vi "DepthSense Acquire.vi"(8 "error in (no error)":errorcluster) -> (0 "error out":errorcluster, 3 "new depth frame":T1)   [LabVIEW 2011]
uses:
  <vilib>/vision/Image Controls.llb/IMAQ Image.ctl
  IT WORKS SO SUCK IT/DepthSense Global Status.vi
  <vilib>/vision/NI_Vision_Development_Module.lvlib
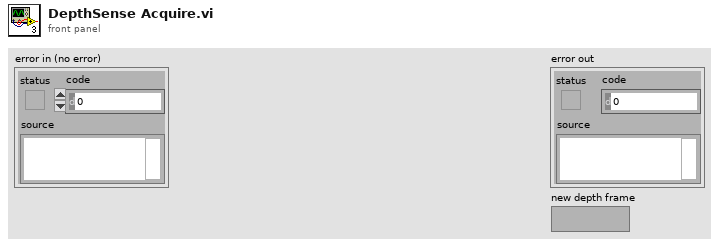
[diagram p1: front panel]
types:
  T1 = typedef "IMAQ Image.ctl" = refnum<image>
  T2 = typedef "Image Type" = u32
  T3 = cluster{"Camera Version":string, "Image Height":i32, "Image Width":i32, "Minimum Framerate":i32, "Maximum Framerate":i32, "Framerate":i32, "Close Mode":bool, "Denoising":bool, "Leakage Algorithm":bool, "Anti-Aliasing":bool, "Camera Status":i32, "API Version":string, "Light Intensity":i32, "Confidence Threshold":u16, "Range":sgl}
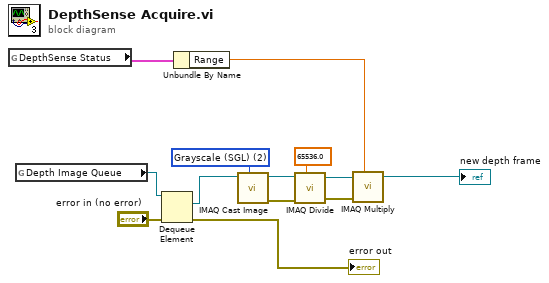
[diagram p0: block diagram]
diagram:
  w9 = T2 2 items=["Grayscale (U8)", "Grayscale (I16)", "Grayscale (SGL)", "Complex (CSG)", "RGB (U32)", "HSL (U32)", "RGB (U64)", "Grayscale (U16)"] ("Image Type")
  n1 = global read "DepthSense Global Status.vi" "DepthSense Status"() -> (w5:T3)
  n2 = global read "DepthSense Global Status.vi" "Depth Image Queue"() -> (w13:refnum<queue>)
  n3 = Dequeue Element(queue=w13, error in (no error)="error in (no error)") -> (element=w10:T1, error out=→"error out":errorcluster)  [unwired: 1 in, 2 out]
  n4 = Unbundle By Name(w5) -> ("Range"=w2:sgl)
  n5 = call "IMAQ Cast Image"("Image Type"=w9, "Image Src"=w10) -> ("error out"=w7:errorcluster, "Image Dst Out"=w8:T1)  [unwired: 8 in]
  n6 = call "IMAQ Divide"("Image Src A"=w8, "Constant"=sgl 65536.0, "error in (no error)"=w7) -> ("Image Dst Out"=w4:T1, "error out"=w3:errorcluster)  [unwired: 4 in]
  n7 = call "IMAQ Multiply"("Image Src A"=w4, "Constant"=w2, "error in (no error)"=w3) -> ("Image Dst Out"=→"new depth frame":T1)  [unwired: 4 in, 1 out]
